vi "draw.vi"(0 "reference":refnum<class "UseCaseNode.lvclass">, 1 "graphics":refnum<class "Graphics.lvclass">, 5 "error in (no error)":errorcluster) -> (14 "reference out":refnum<class "UseCaseNode.lvclass">, 19 "error out":errorcluster)   [LabVIEW 2016, in "UseCaseNode.lvclass"]
doc: "public void draw(Graphics2D g2, Point2D p, Point2D q)"
uses:
  <resource>/Framework/Providers/Open_GDS/UML/UseCaseNode_class/UseCaseNode.lvclass
  C:/Program Files (x86)/National Instruments/LabVIEW 2016/resource/Framework/Providers/Open_GDS/UML/RectangularNode_class/RectangularNode.lvclass
  <resource>/Framework/Providers/Open_GDS/UML/Graphics_class/Graphics.lvclass
  <resource>/Framework/Providers/Open_GDS/UML/MultiLineString_class/MultiLineString.lvclass
  <resource>/Framework/Providers/Open_GDS/UML/RectangularNode_class/RectangularNode.lvclass
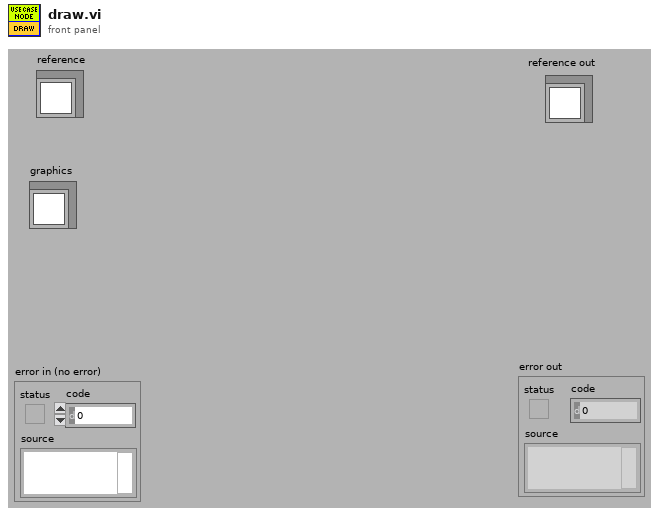
[diagram p1: front panel]
types:
  T1 = typedef "UseCaseNode.lvclass/ObjectAttributes.ctl" = cluster{"name":refnum<class "MultiLineString.lvclass">, "DEFAULT_WIDTH":i32, "DEFAULT_HEIGHT":i32}
  T2 = typedef "RectangularNode.lvclass/ObjectAttributes.ctl" = cluster{"bounds":T3}
  T3 = typedef "Rectangle Rectangle2D.ctl" = cluster{"x":dbl, "y":dbl, "width":dbl, "height":dbl}
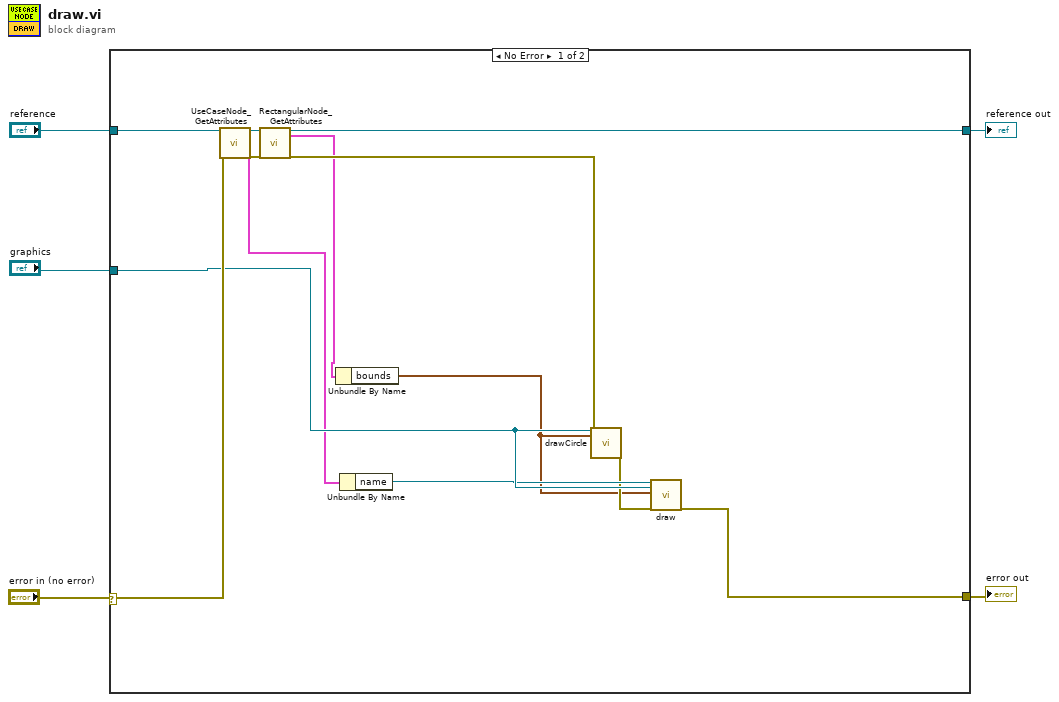
[diagram p0: block diagram]
diagram:
  n1 = case shown="No Error" "error in (no error)" {
    selector: "error in (no error)" -> [w16 w19]
    tunnel: "reference" -> [w18 w20]
    tunnel: [w17 w19] -> w4
    tunnel: [w7 w20] -> w3
    tunnel: "graphics" -> [w15 _]
    frame No Error {
      n2 = call <resource>:"UseCaseNode_GetAttributes.vi"("reference in"=w18, "error in (no error)"=w16) -> ("reference out"=w10:refnum<class "UseCaseNode.lvclass">, "Data"=w11:T1, "error out"=w9:errorcluster)  [unwired: 1 in, 14 out]
      n3 = call <resource>:"RectangularNode_GetAttributes.vi"("reference in"=w10, "error in (no error)"=w9) -> ("reference out"=w7:refnum<class "UseCaseNode.lvclass">, "Data"=w6:T2, "error out"=w8:errorcluster)  [unwired: 14 in, 1 out]
      n4 = Unbundle By Name(w6) -> ("bounds"=w12:T3)
      n5 = Unbundle By Name(w11) -> ("name"=w14:refnum<class "MultiLineString.lvclass">)
      n6 = call-dynamic "drawCircle.vi"("reference"=w15, "rectangle"=w12, "error in (no error)"=w8) -> ("error out"=w13:errorcluster)  [unwired: 15 in, 1 out]
      n7 = call-dynamic "draw.vi"("reference"=w14, "graphics"=w15, "bounds"=w12, "error in (no error)"=w13) -> ("error out"=w17:errorcluster)  [unwired: 14 in, 1 out]
    }
    frame Error {
    }
  }
  "reference out" <- w3
  "error out" <- w4
